vi "Obtain Request Events.vi"(8 "error in":errorcluster, 10 "Create New? (F)":bool) -> (0 "error out":errorcluster, 2 "Mensajes Request Events":T1)   [LabVIEW 2019, in "Mensajes.lvlib"]
doc: "This VI Obtains/Creates the Requests events that will be used for other modules to communicate with the module that owns this VI. These Requests events will be accessed only via Public API methods for this module.\n\n<b>NOTE</b>: The contents of this VI are automatically generated and modified by the <b>Tools > DQMH Consortium > DQMH</b> utilities. Consider using those utilities instead of making your own modifications to this VI.\n_____\nBased on DQMH Dev Tools: Project Template 7.1.0.1503."
uses:
  Mensajes.lvlib
  Request Events--cluster.ctl
  Stop Argument--cluster.ctl
  Show Panel Argument--cluster.ctl
  Hide Panel Argument--cluster.ctl
  Show Diagram Argument--cluster.ctl
  Get Module Execution Status Argument--cluster.ctl
  Draw FP in Subpanel Argument--cluster.ctl
  Remove From Subpanel Argument--cluster.ctl
  Display Message Argument--cluster.ctl
  Set Display Style Argument--cluster.ctl
panel:
  # "NOTE: The contents of this VI are automatically generated and modified by the Tools > DQMH Consortium > DQMH utilities. Consider using those utilities instead of making your own modifications to this VI."
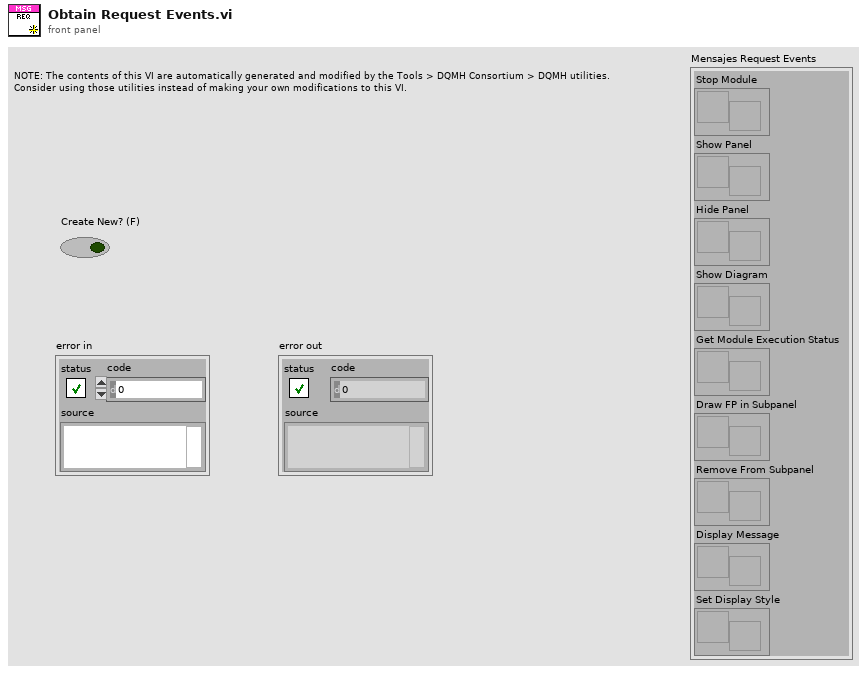
[diagram p1: front panel]
types:
  T1 = typedef "Mensajes.lvlib/Request Events--cluster.ctl" = cluster{"Stop Module":refnum<user-event>, "Show Panel":refnum<user-event>, "Hide Panel":refnum<user-event>, "Show Diagram":refnum<user-event>, "Get Module Execution Status":refnum<user-event>, "Draw FP in Subpanel":refnum<user-event>, "Remove From Subpanel":refnum<user-event>, "Display Message":refnum<user-event>, "Set Display Style":refnum<user-event>}
  T2 = typedef "Mensajes.lvlib/Set Display Style Argument--cluster.ctl" = cluster{"Module ID":i32, "Display Style":enum16{"Normal", "Backslash", "Password", "Hexadecimal"}}
  T3 = typedef "Mensajes.lvlib/Display Message Argument--cluster.ctl" = cluster{"Module ID":i32, "Message":string}
  T4 = typedef "Mensajes.lvlib/Remove From Subpanel Argument--cluster.ctl" = cluster{"Module ID":i32, "Boolean":bool}
  T5 = typedef "Mensajes.lvlib/Draw FP in Subpanel Argument--cluster.ctl" = cluster{"Module ID":i32, "Sub Panel":refnum<vi>}
  T6 = typedef "Mensajes.lvlib/Get Module Execution Status Argument--cluster.ctl" = cluster{"Module ID":i32, "Running?":bool}
  T7 = typedef "Mensajes.lvlib/Show Diagram Argument--cluster.ctl" = cluster{"Module ID":i32, "Debug?":bool}
  T8 = typedef "Mensajes.lvlib/Show Panel Argument--cluster.ctl" = cluster{"Module ID":i32, "Show Panel?":bool}
  T9 = typedef "Mensajes.lvlib/Hide Panel Argument--cluster.ctl" = cluster{"Module ID":i32, "Hide Panel?":bool}
  T10 = typedef "Mensajes.lvlib/Stop Argument--cluster.ctl" = cluster{"Module ID":i32, "Origin":string, "Exit via Stop Module Req?":bool, "Wait for Module to stop?":bool}
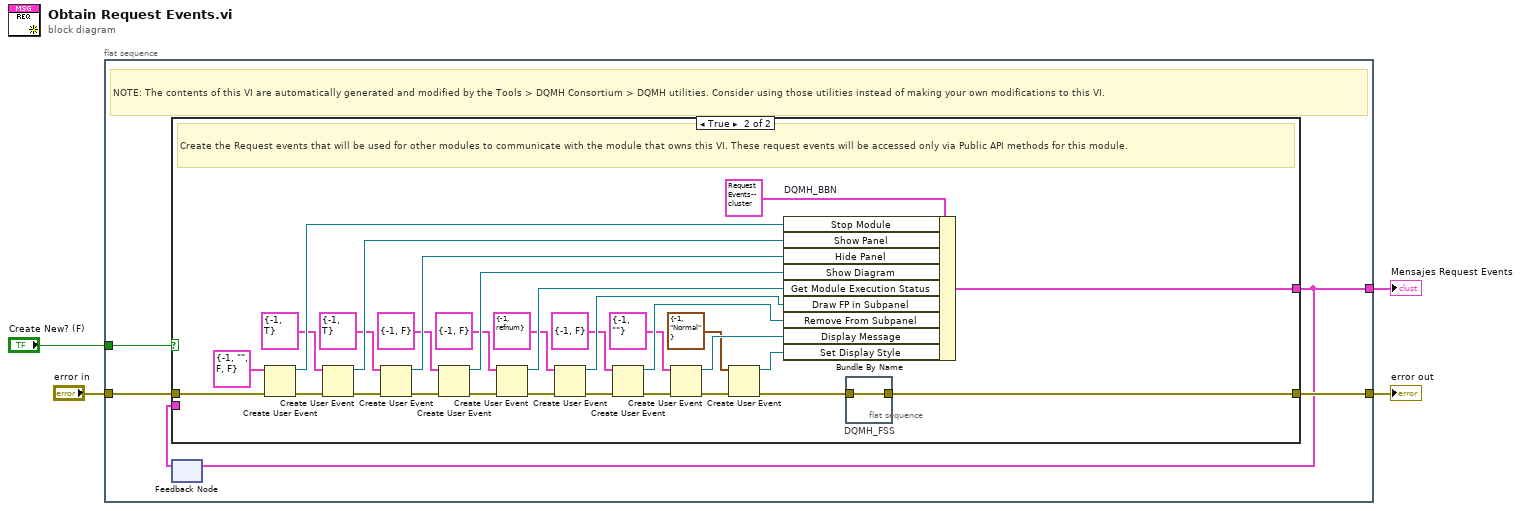
[diagram p0: block diagram]
diagram:
  n1 = flat-sequence {
    tunnel: [w9] -> w4
    tunnel: "error in" -> [w8]
    tunnel: [w6] -> w2
    tunnel: "Create New? (F)" -> [w5]
    frame #0 {
      # "NOTE: The contents of this VI are automatically generated and modified by the Tools > DQMH Consortium > DQMH utilities. Consider using those utilities instead of making your own modifications to this VI."
      n2 = feedback #1() -> (w7:T1)  [unwired: 1 in]
      n3 = case shown="True" w5 {
        tunnel: [w10 w30] -> w9
        tunnel: w8 -> [w10 w42]
        tunnel: [w11 w39] -> w6
        tunnel: w7 -> [w11 _]
        frame False {
        }
        frame True {
          # "Create the Request events that will be used for other modules to communicate with the module that owns this VI. These request events will be accessed only via Public API methods for this module."
          n4 = Create User Event(user event datatype=T10 {"Module ID"=-1, "Origin"="", "Exit via Stop Module Req?"=FALSE, "Wait for Module to stop?"=FALSE} ("Stop Argument"), error in=w42) -> (user event=w40:refnum<user-event>, error out=w37:errorcluster)
          n5 = Create User Event(user event datatype=T8 {"Module ID"=-1, "Show Panel?"=TRUE} ("Show Panel Argument"), error in=w37) -> (user event=w36:refnum<user-event>, error out=w34:errorcluster)
          n6 = Create User Event(user event datatype=T9 {"Module ID"=-1, "Hide Panel?"=TRUE} ("Hide Panel"), error in=w34) -> (user event=w33:refnum<user-event>, error out=w32:errorcluster)
          n7 = Create User Event(user event datatype=T7 {"Module ID"=-1, "Debug?"=FALSE} ("Show Diagram Argument"), error in=w32) -> (user event=w28:refnum<user-event>, error out=w29:errorcluster)
          n8 = Create User Event(user event datatype=T6 {"Module ID"=-1, "Running?"=FALSE} ("Get Module Execution Status Argument"), error in=w29) -> (user event=w25:refnum<user-event>, error out=w26:errorcluster)
          n9 = Create User Event(user event datatype=T5 {"Module ID"=-1, "Sub Panel"=refnum} ("Draw FP in Subpanel Argument"), error in=w26) -> (user event=w22:refnum<user-event>, error out=w23:errorcluster)
          n10 = Create User Event(user event datatype=T4 {"Module ID"=-1, "Boolean"=FALSE} ("Remove From Subpanel Argument"), error in=w23) -> (user event=w19:refnum<user-event>, error out=w20:errorcluster)
          n11 = Create User Event(user event datatype=T3 {"Module ID"=-1, "Message"=""} ("Display Message Argument"), error in=w20) -> (user event=w16:refnum<user-event>, error out=w17:errorcluster)
          n12 = Create User Event(user event datatype=T2 {"Module ID"=-1, "Display Style"=enum."Normal"} ("Set Display Style Argument"), error in=w17) -> (user event=w13:refnum<user-event>, error out=w14:errorcluster)
          n13 = Bundle By Name "DQMH_BBN"(cluster=T1 {"Stop Module"=refnum, "Show Panel"=refnum, "Hide Panel"=refnum, "Show Diagram"=refnum, "Get Module Execution Status"=refnum, "Draw FP in Subpanel"=refnum, "Remove From Subpanel"=refnum, "Display Message"=refnum, "Set Display Style"=refnum} ("output cluster"), "Stop Module"=w40, "Show Panel"=w36, "Hide Panel"=w33, "Show Diagram"=w28, "Get Module Execution Status"=w25, "Draw FP in Subpanel"=w22, "Remove From Subpanel"=w19, "Display Message"=w16, "Set Display Style"=w13) -> (w39:T1)
          n14 = flat-sequence "DQMH_FSS" {
            tunnel: w14 -> [w43]
            tunnel: [w43] -> w30
            frame #0 {
            }
          }
        }
      }
      n15 = feedback-in #1(w6) -> ()
    }
  }
  "Mensajes Request Events" <- w2
  "error out" <- w4
